vi "XNET Device Property Node.vi"   [LabVIEW 2018]
doc: "Property node used to read/write properties for an XNET Device I/O name."
uses:
  <resource>/objmgr/xnet.rc
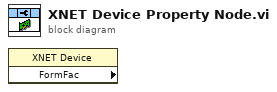
[diagram p0: block diagram]
diagram:
  n1 = property class="XNET Device" props=["FormFac"]() -> ()  [unwired: 2 in, 3 out]
